vi "Count Size Matches.vi"(8 "error in":errorcluster, 10 "Expected Size in":i32, 11 "Sizes":i32[](array[numeric])) -> (0 "% of Daily Expected Good":string, 1 "% Good":string, 2 "Daily SBD Messages (IMEI Match)":string, 3 "Missed Tx (IMEI Match)":string, 4 "error out":errorcluster)   [LabVIEW 2014]
panel:
  out "Daily SBD Messages (IMEI Match)":i32
  out "Missed Tx (IMEI Match)":i32
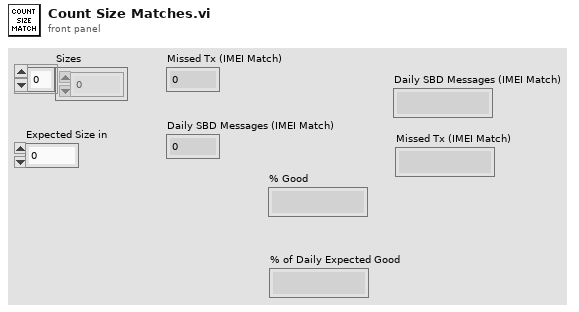
[diagram p1: front panel]
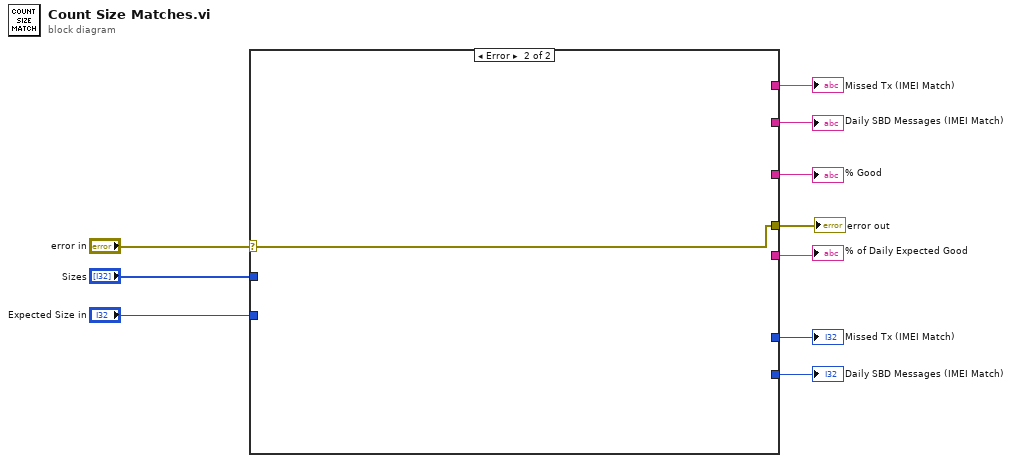
[diagram p0: block diagram]
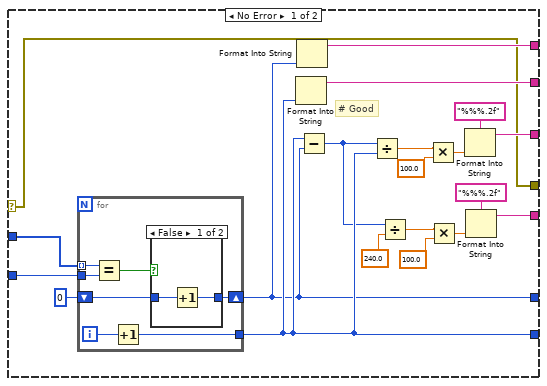
[diagram p2: hidden frame]
diagram:
  n1 = case shown="Error" "error in" {
    selector: "error in" -> [w11 w41]
    tunnel: "Expected Size in" -> [w29 _]
    tunnel: "Sizes" -> [w28 _]
    tunnel: [w27 _] -> w8
    tunnel: [w26 _] -> w7
    tunnel: [w25 _] -> w6
    tunnel: [w24 _] -> w5
    tunnel: [w19 _] -> w4
    tunnel: [w18 _] -> w3
    tunnel: [w11 w41] -> w1
    frame No Error {
      # "# Good"
      n2 = for {
        tunnel: w28 -> [w34] mode=indexing
        tunnel: w29 -> [w35]
        tunnel: [w36] -> w25
        shift-right: [w31] -> w24
        shift-left: 0 ("Expected Size") -> [w32]
        i -> [w37]
        n3 = Equal?(x=w34, y=w35) -> (x = y?=w33:bool)
        n4 = Increment(x=w37) -> (x+1=w36:i32)
        n5 = case shown="False" w33 {
          tunnel: w32 -> [w38 w40]
          tunnel: [w39 w40] -> w31
          frame False {
            n6 = Increment(x=w38) -> (x+1=w39:i32)
          }
          frame True {
          }
        }
      }
      n7 = Format Into String(w25) -> (resulting string=w26:string)  [unwired: 3 in, 1 out]
      n8 = Format Into String(w24) -> (resulting string=w27:string)  [unwired: 3 in, 1 out]
      n9 = Subtract(x=w25, y=w24) -> (x-y=w12:i32)
      n10 = Divide(x=w12, y=w25) -> (x/y=w23:dbl)
      n11 = Divide(x=w12, y=240.0) -> (x/y=w14:dbl)
      n12 = Multiply(x=w23, y=100.0) -> (x*y=w21:dbl)
      n13 = Multiply(x=w14, y=100.0) -> (x*y=w16:dbl)
      n14 = Format Into String(format string="%%%.2f", w21) -> (resulting string=w19:string)  [unwired: 2 in, 1 out]
      n15 = Format Into String(format string="%%%.2f", w16) -> (resulting string=w18:string)  [unwired: 2 in, 1 out]
    }
    frame Error {
    }
  }
  "Missed Tx (IMEI Match)" <- w5
  "Daily SBD Messages (IMEI Match)" <- w6
  "Missed Tx (IMEI Match)" <- w8
  "Daily SBD Messages (IMEI Match)" <- w7
  "% Good" <- w4
  "% of Daily Expected Good" <- w3
  "error out" <- w1
